vi "Set Bucket Website Configuration.vi"(7 "Website Configuration":T1={"IndexDocument"={"Suffix"="index.html"}, "ErrorDocument"={"Key"="404.html"}}, 8 "error in (no error)":errorcluster, 9 "Bucket":string) -> (0 "error out":errorcluster)   [LabVIEW 2011, in "LV Interface for Amazon S3.lvlib"]
doc: "This operation <B>sets the website configuration</B>. This operation <B>requires the S3:PutBucketWebsite permission</B>. By default, <B>only the bucket owner can configure the website attached to a bucket</B>. However, bucket <B>owners can allow other users to set the website configuration by</B> writing a bucket policy <B>granting them the S3:PutBucketWebsite permission</B>."
uses:
  LV Interface for Amazon S3.lvlib
  Typedefs/AMZ_S3_API_WebsiteConfiguration.ctl
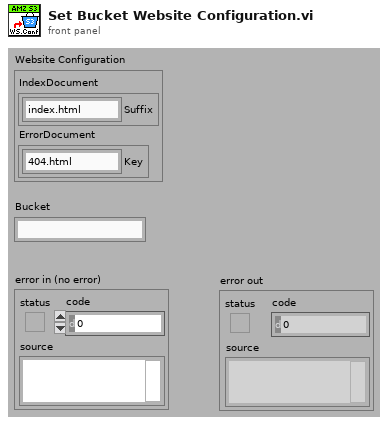
[diagram p1: front panel]
types:
  T1 = typedef "LV Interface for Amazon S3.lvlib/AMZ_S3_API_WebsiteConfiguration.ctl" = cluster{"IndexDocument":cluster{"Suffix":string}, "ErrorDocument":cluster{"Key":string}}
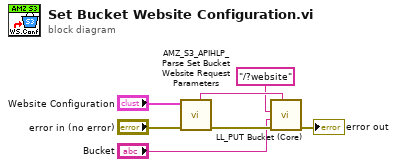
[diagram p0: block diagram]
diagram:
  n1 = call "AMZ_S3_APIHLP_Parse Set Bucket Website Request Parameters.vi"("error in (no error)"="error in (no error)", "Website Configuration"="Website Configuration") -> ("error out"=w5:errorcluster, "PUT Data"=w4:string)  [unwired: 8 in]
  n2 = call "LL_PUT Bucket (Core).vi"("Data"=w4, "error in (no error)"=w5, "Bucket"="Bucket", "Path and query string"="/?website") -> ("error out"=→"error out":errorcluster)  [unwired: 4 in, 3 out]
